vi "String.Add an Indexed Name list to Variant Attributes.vi"(10 "Name List":string[](array[string]), 11 "Variant":variant) -> (3 "Variant Out":variant)   [LabVIEW 2019]
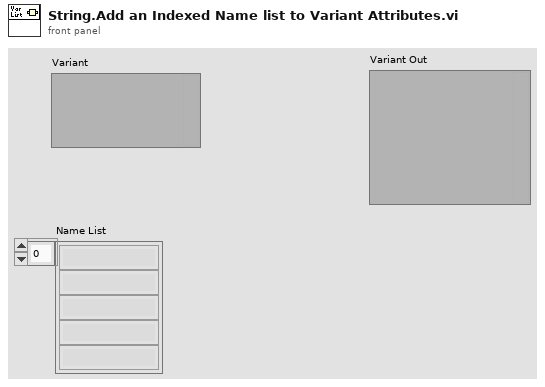
[diagram p1: front panel]
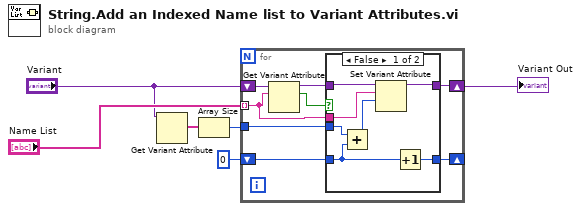
[diagram p0: block diagram]
diagram:
  n1 = Get Variant Attribute(Variant="Variant") -> (names=w6:string[])  [unwired: 3 in, 3 out]
  n2 = Array Size(array=w6) -> (size(s)=w5:i32)
  n3 = for {
    tunnel: "Name List" -> [w7] mode=indexing
    tunnel: w5 -> [w10]
    shift-right: [w9] -> _
    shift-left: 0 -> [w11]
    shift-right: [w8] -> w1
    shift-left: "Variant" -> [w14]
    n4 = Get Variant Attribute(Variant=w14, name=w7) -> (duplicate Variant=w13:variant, found=w12:bool)  [unwired: 2 in, 2 out]
    n5 = case shown="False" w12 {
      tunnel: w13 -> [w19 w22]
      tunnel: w11 -> [w16 w23]
      tunnel: w10 -> [w17 _]
      tunnel: [w21 w23] -> w9
      tunnel: [w20 w22] -> w8
      tunnel: w7 -> [w18 _]
      frame False {
        n6 = Add(x=w17, y=w16) -> (x+y=w15:i32)
        n7 = Set Variant Attribute(Variant=w19, name=w18, value=w15) -> (Variant out=w20:variant)  [unwired: 1 in, 2 out]
        n8 = Increment(x=w16) -> (x+1=w21:i32)
      }
      frame True {
        # "Do Nothing"
      }
    }
  }
  "Variant Out" <- w1
